vi "Set Minimal Maximal Size.vi"(4 "Vertical":cluster{"Minimal":i16, "Maximal":i16}={"Minimal"=0, "Maximal"=32767}, 6 "Horizontal":cluster{"Minimal":i16, "Maximal":i16}={"Minimal"=0, "Maximal"=32767}, 8 "error in (no error)":errorcluster, 11 "MMI Scaling in":refnum<class "IObject.lvclass">) -> (0 "error out":errorcluster, 3 "MMI Scaling out":refnum<class "IObject.lvclass">)   [LabVIEW 2021, in "IObject.lvclass"]
uses:
  IObject.lvclass
  IObject.lvclass/IObject.ctl
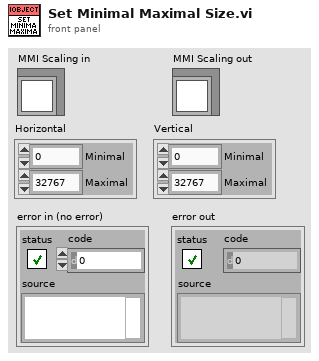
[diagram p1: front panel]
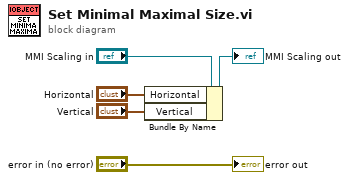
[diagram p0: block diagram]
diagram:
  n1 = Bundle By Name(cluster="MMI Scaling in", "Horizontal"="Horizontal", "Vertical"="Vertical") -> (→"MMI Scaling out":refnum<class "IObject.lvclass">)
  "error out" <- "error in (no error)"
